vi "Test_program.vi"() -> ()   [LabVIEW 2015]
uses:
  Control_card.lvclass
panel:
  out "Waveform Graph":dbl[](graph)
  in  "Start":dbl
  out "Progress":string
  out "error out":errorcluster
  in  "error in":errorcluster
  in  "Acquisition":T1={"Sample Rate"=6000000000.0, "Clock mode"=enum."Internal", "Mode"=0, "Depth"=816000.0, "Segment Size"=816000.0, "Trigger Timeout"=1000000.0, "Trigger Holdoff"=0.0, "Trigger Delay"=0.0} {"Mode" items=["Single", "Dual", "Quad", "Octal"]}
  in  "Trigger":T2={"Slope"=0, "Level"=30, "Source"=0, "External Range"=2000, "External Coupling"=0, "External"=TRUE, "Disable"=FALSE, "External Impedance"=1} {"Slope" items=["Rising", "Falling"]; "External Coupling" items=["DC", "AC"]; "External Impedance" items=["50 Ohm", "HiZ"]}
  in  "Channel":T3={"Coupling"=0, "Differential Input"=FALSE, "Direct-to-ADC"=FALSE, "Range"=2000, "Impedance"=50, "DC Offset"=0, "Filter"=0} {"Impedance" min=50 max=1000000 step=999950; "Coupling" items=["DC", "AC"]}
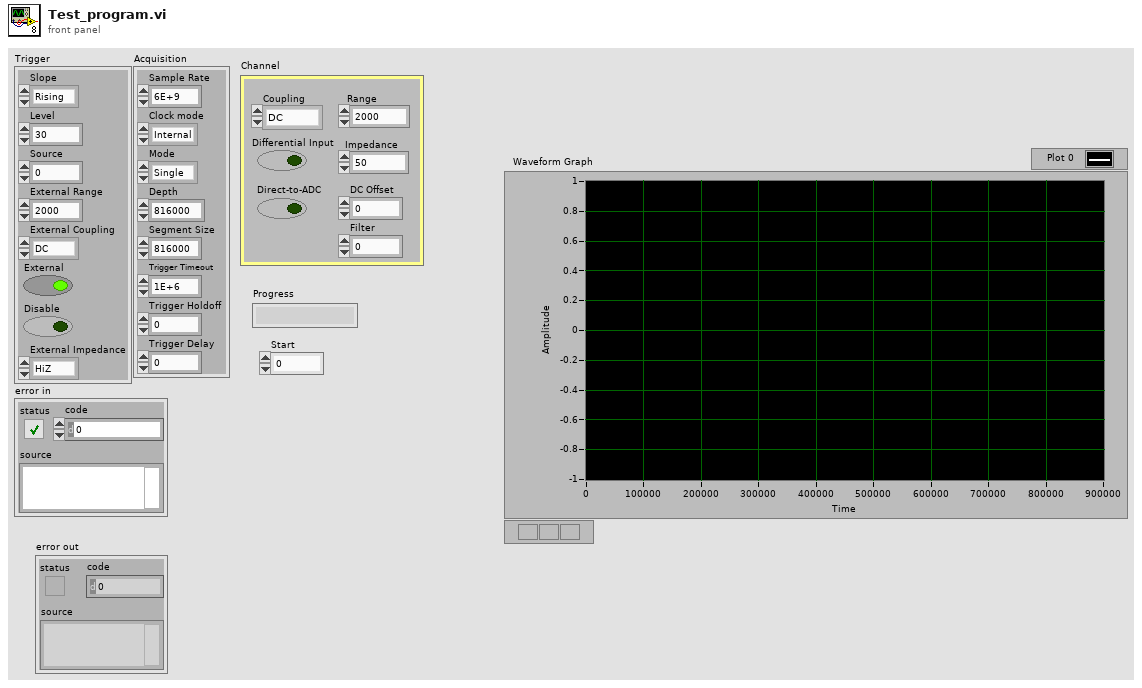
[diagram p1: front panel]
types:
  T1 = cluster{"Sample Rate":dbl, "Clock mode":enum16{"Internal", "External", "Reference"}, "Mode":u16, "Depth":dbl, "Segment Size":dbl, "Trigger Timeout":dbl, "Trigger Holdoff":dbl, "Trigger Delay":dbl}
  T2 = cluster{"Slope":u16, "Level":i32, "Source":i32, "External Range":u32, "External Coupling":u16, "External":bool, "Disable":bool, "External Impedance":u16}
  T3 = cluster{"Coupling":u16, "Differential Input":bool, "Direct-to-ADC":bool, "Range":u32, "Impedance":u32, "DC Offset":i32, "Filter":i32}
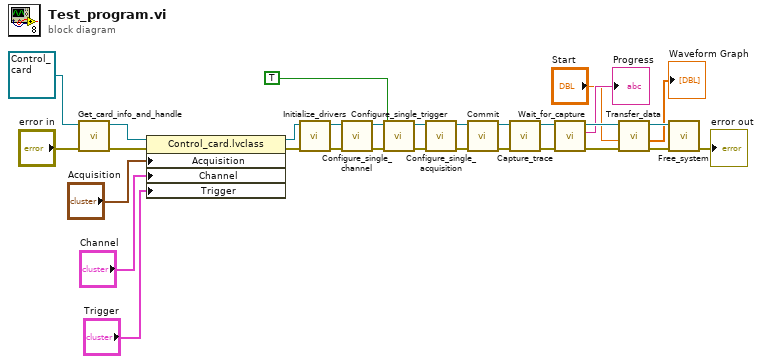
[diagram p0: block diagram]
diagram:
  n1 = call "Get_card_info_and_handle.vi"("error in (no error)"="error in", "Initialize_card in"=refnum<class "Control_card.lvclass"> refnum ("Initialize_card.lvclass")) -> ("error out"=w22:errorcluster, "Initialize_card out"=w29:refnum<class "Control_card.lvclass">)  [unwired: 8 in]
  n2 = property class="Control_card.lvclass"(reference=w29, error in=w22, "Acquisition"="Acquisition", "Channel"="Channel", "Trigger"="Trigger") -> (reference out=w25:refnum<class "Control_card.lvclass">, error out=w24:errorcluster)
  n3 = call-dynamic "Initialize_drivers.vi"("error in (no error)"=w24, "Initialize_card in"=w25) -> ("error out"=w20:errorcluster, "Initialize_card out"=w21:refnum<class "Control_card.lvclass">)  [unwired: 8 in]
  n4 = call-dynamic "Configure_single_channel.vi"("error in (no error)"=w20, "Initialize_card in"=w21) -> ("error out"=w18:errorcluster, "Initialize_card out"=w19:refnum<class "Control_card.lvclass">)  [unwired: 8 in]
  n5 = call-dynamic "Configure_single_trigger.vi"("error in (no error)"=w18, "Enable Trigger?"=TRUE, "Initialize_card in"=w19) -> ("error out"=w16:errorcluster, "Initialize_card out"=w17:refnum<class "Control_card.lvclass">)  [unwired: 7 in]
  n6 = call-dynamic "Configure_single_acquisition.vi"("error in (no error)"=w16, "Initialize_card in"=w17) -> ("error out"=w14:errorcluster, "Initialize_card out"=w15:refnum<class "Control_card.lvclass">)  [unwired: 8 in]
  n7 = call-dynamic "Commit.vi"("error in (no error)"=w14, "Initialize_card in"=w15) -> ("error out"=w6:errorcluster, "Initialize_card out"=w7:refnum<class "Control_card.lvclass">)  [unwired: 8 in]
  n8 = call-dynamic "Capture_trace.vi"("error in (no error)"=w6, "Initialize_card in"=w7) -> ("error out"=w4:errorcluster, "Initialize_card out"=w5:refnum<class "Control_card.lvclass">)  [unwired: 8 in]
  n9 = call-dynamic "Wait_for_capture.vi"("error in (no error)"=w4, "Initialize_card in"=w5) -> ("error out"=w12:errorcluster, "Progress"=→"Progress":string, "Initialize_card out"=w13:refnum<class "Control_card.lvclass">)  [unwired: 6 in]
  n10 = call-dynamic "Transfer_data.vi"("error in (no error)"=w12, "Start"="Start", "Initialize_card in"=w13) -> ("error out"=w9:errorcluster, "Data in Volts"=→"Waveform Graph":dbl[], "Initialize_card out"=w10:refnum<class "Control_card.lvclass">)  [unwired: 6 in]
  n11 = call-dynamic "Free_system.vi"("error in (no error)"=w9, "Initialize_card in"=w10) -> ("error out"=→"error out":errorcluster)  [unwired: 8 in, 1 out]
